vi "execute_adapters.vi"(8 "error in (no error)":errorcluster, 11 "GenericTrajectory in":refnum<class "GenericTrajectory.lvclass">) -> (0 "error out":errorcluster, 3 "GenericTrajectory out":refnum<class "GenericTrajectory.lvclass">)   [LabVIEW 2010, in "GenericTrajectory.lvclass"]
doc: "executes the adapter to the ImageAssembler; can be overridden to execute any further adapters"
uses:
  GenericTrajectory.lvclass
  common/classes/ErrorController/ErrorController/class_data.vi
  common/classes/GenericComponent/GenericComponent/GenericComponent.lvclass
  ImageAssembler/GenericImageAssembler/GenericImageAssembler/GenericImageAssembler.lvclass
  Adapter/GenericAdapter/GenericAdapter/GenericAdapter.lvclass
  common/classes/ErrorController/ErrorController/ErrorController.lvclass
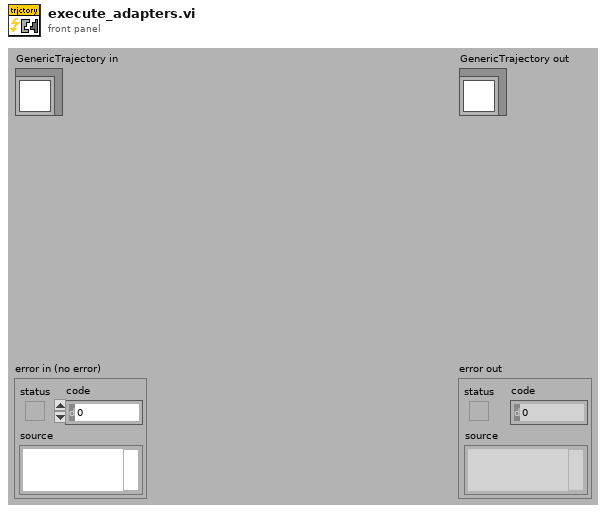
[diagram p1: front panel]
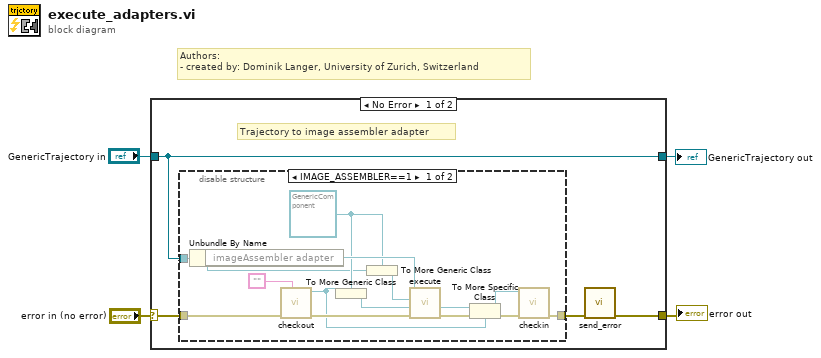
[diagram p0: block diagram]
diagram:
  # "Authors: \n- created by: Dominik Langer, University of Zurich, Switzerland"
  n1 = case shown="No Error" "error in (no error)" {
    selector: "error in (no error)" -> [w8 w25]
    tunnel: [w5 w25] -> w1
    tunnel: [w7 w24] -> w4
    tunnel: "GenericTrajectory in" -> [w7 w24]
    frame No Error {
      # "Trajectory to image assembler adapter"
      n2 = disable-structure shown="IMAGE_ASSEMBLER==1" {
        disable-tunnel: [w22 w23] -> w6
        disable-tunnel: w8 -> [w21 w23]
        disable-tunnel: w7 -> [w10 _]
        frame condition #0 {
          w17 = refnum<class "GenericComponent.lvclass"> refnum ("GenericPlugin.lvclass")
          n3 = Unbundle By Name(w10) -> ("imageAssembler adapter"=w20:refnum<class "GenericAdapter.lvclass">)
          n4 = call "checkout.vi"("locked by?"="", "error in (no error)"=w21) -> ("error out"=w18:errorcluster, "GenericImageAssembler out"=w11:refnum<class "GenericImageAssembler.lvclass">)  [unwired: 8 in]
          n5 = To More Generic Class(target class=w17, reference=w11) -> (generic class reference=w16:refnum<class "GenericComponent.lvclass">)
          n6 = To More Generic Class(target class=w17, reference=w10) -> (generic class reference=w19:refnum<class "GenericComponent.lvclass">)
          n7 = call-dynamic "execute.vi"("error in (no error)"=w18, "B in"=w16, "A in"=w19, "GenericAdapter in"=w20) -> ("error out"=w15:errorcluster, "B out"=w14:refnum<class "GenericComponent.lvclass">)  [unwired: 6 out]
          n8 = To More Specific Class(target class=w11, reference=w14, error in=w15) -> (specific class reference=w12:refnum<class "GenericImageAssembler.lvclass">, error out=w13:errorcluster)
          n9 = call-dynamic "checkin.vi"("error in (no error)"=w13, "GenericImageAssembler in"=w12) -> ("error out"=w22:errorcluster)  [unwired: 8 in, 1 out]
        }
        frame condition #1 (active) {
        }
      }
      n10 = call "send_error.vi"("error in (no error)"=w6) -> ("error out"=w5:errorcluster)  [unwired: 10 in]
    }
    frame Error {
    }
  }
  "error out" <- w1
  "GenericTrajectory out" <- w4
